vi "Read Configuration File Path.vi"(8 "Error In":errorcluster, 11 "CS++RTRootActor in":refnum<class "CS++RTRootActor.lvclass">) -> (0 "Error Out":errorcluster, 2 "Configuration File Path":path=path "C:/CSPP-RT.ini", 3 "CS++RTRootActor out":refnum<class "CS++RTRootActor.lvclass">)   [LabVIEW 2014, in "CS++RTRoot.lvlib" / "CS++RTRootActor.lvclass"]
doc: "Read configuration file path from attribute."
uses:
  CS++RTRootActor.lvclass
  CS++RTRootActor.lvclass/CS++RTRootActor.ctl
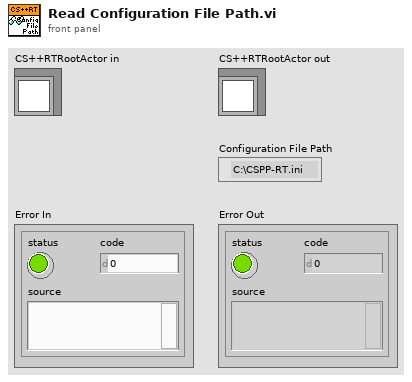
[diagram p1: front panel]
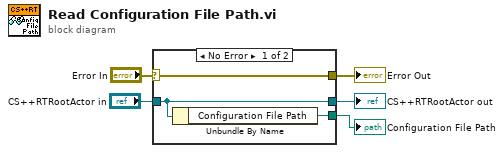
[diagram p0: block diagram]
diagram:
  n1 = case shown="No Error" "Error In" {
    selector: "Error In" -> [w8 w9]
    tunnel: [w8 w9] -> w4
    tunnel: [w7 w10] -> w2
    tunnel: "CS++RTRootActor in" -> [w7 w10]
    tunnel: [w6 _] -> w1
    frame No Error {
      n2 = Unbundle By Name(w7) -> ("Configuration File Path"=w6:path)
    }
    frame Error {
    }
  }
  "Error Out" <- w4
  "CS++RTRootActor out" <- w2
  "Configuration File Path" <- w1
